vi "ConvertStatusRegistersToSystemStatusArray.vi"(0 "Array of StatusRegister":T1[](array[typedef]), 5 "error in":errorcluster) -> (14 "Array of SystemStatus":T2[](array[typedef]), 19 "error out":errorcluster)   [LabVIEW 2026]
uses:
  GeneralCommands/SystemStatus.ctl
  GeneralCommands/Status.ctl
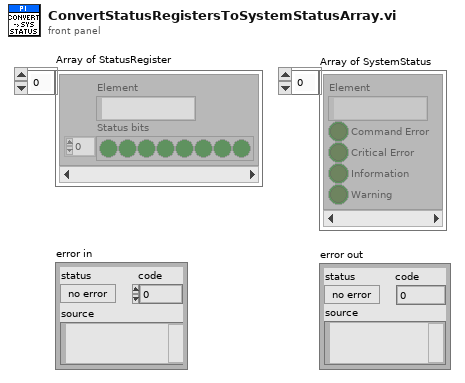
[diagram p1: front panel]
types:
  T1 = typedef "Status.ctl" = cluster{"Element":string, "Status bits":bool[]}
  T2 = typedef "SystemStatus.ctl" = cluster{"Element":string, "Command Error":bool, "Critical Error":bool, "Information":bool, "Warning":bool}
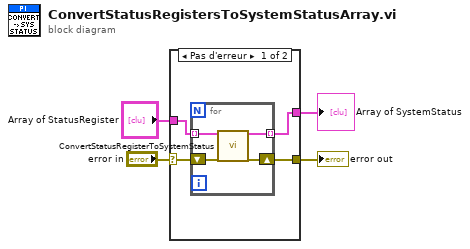
[diagram p0: block diagram]
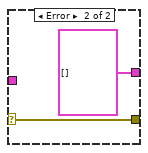
[diagram p2: hidden frame]
diagram:
  n1 = case shown="Pas d'erreur" "error in" {
    selector: "error in" -> [w7 w14]
    tunnel: [w8 w14] -> w3
    tunnel: [w6 T2[] []] -> w2
    tunnel: "Array of StatusRegister" -> [w5 _]
    frame No Error {
      n2 = for {
        shift-right: [w12] -> w8
        shift-left: w7 -> [w10]
        tunnel: [w11] -> w6 mode=indexing
        tunnel: w5 -> [w9] mode=indexing
        n3 = call "ConvertStatusRegisterToSystemStatus.vi"("Status"=w9, "error in"=w10) -> ("SystemStatus"=w11:T2, "error out"=w12:errorcluster)  [unwired: 16 in]
      }
    }
    frame Error {
    }
  }
  "error out" <- w3
  "Array of SystemStatus" <- w2
